vi "Get_Order.vi"(1 "Control in":T1={"queue"=refnum, "error"={"status"=FALSE, "code"=0, "source"=""}, "Step"={"Name"="", "Timeout"=0.0}, "Algorythm"=[{"Name"="Init", "Timeout"=0.0}]}) -> (13 "timed out?":bool, 15 "Control out":T1={"queue"=refnum, "error"={"status"=FALSE, "code"=0, "source"=""}, "Step"={"Name"="", "Timeout"=0.0}, "Algorythm"=[{"Name"="Init", "Timeout"=0.0}]})   [LabVIEW 2023, in "SFC.lvlib"]
uses:
  SFC.lvlib
  TypeDef/Control TypeDef.ctl
  TypeDef/Step TypeDef.ctl
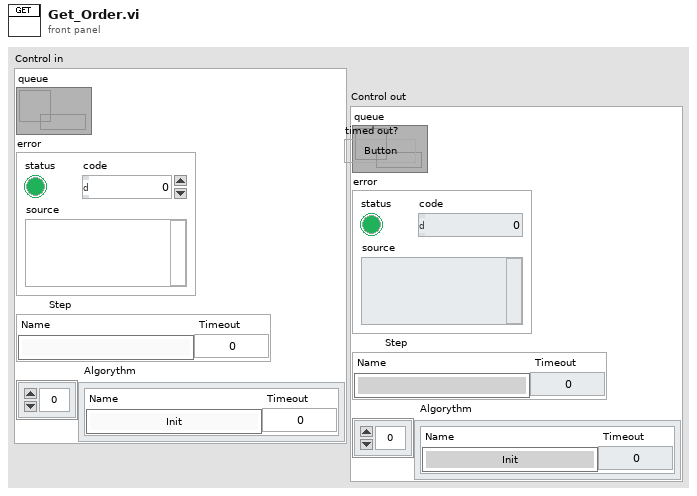
[diagram p1: front panel]
types:
  T1 = typedef "SFC.lvlib/Control TypeDef.ctl" = cluster{"queue":refnum<queue>, "error":errorcluster, "Step":T2, "Algorythm":T2[]}
  T2 = typedef "SFC.lvlib/Step TypeDef.ctl" = cluster{"Name":string, "Timeout":dbl}
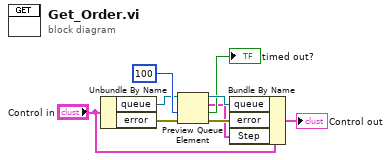
[diagram p0: block diagram]
diagram:
  n1 = Unbundle By Name("Control in") -> ("queue"=w8:refnum<queue>, "error"=w7:errorcluster)
  n2 = Preview Queue Element(queue=w8, timeout in ms (-1)=100, error in (no error)=w7) -> (queue out=w4:refnum<queue>, element=w1:T2, timed out?=→"timed out?":bool, error out=w3:errorcluster)
  n3 = Bundle By Name(cluster="Control in", "queue"=w4, "error"=w3, "Step"=w1) -> (→"Control out":T1)
